vi "ComputeACPadPositions.vi"(0 "Theta Calibration":dbl format="%#_8g", 1 "X cp":dbl format="%#_8g", 2 "Y cp":dbl format="%#_8g", 3 "Stage Initial\nRotation":dbl, 4 "Sensor Path":path=path "R0Hamamatsu.txt ") -> ()   [LabVIEW 2018]
uses:
  <vilib>/Analysis/coordinate.llb/2D Cartesian Coordinate Rotation (Scalar).vi
  <vilib>/Utility/file.llb/Read Delimited Spreadsheet (DBL).vi
  <vilib>/Utility/file.llb/Write Delimited Spreadsheet (DBL).vi
  <vilib>/Analysis/NI_AALPro.lvlib
panel:
  out "error out":errorcluster
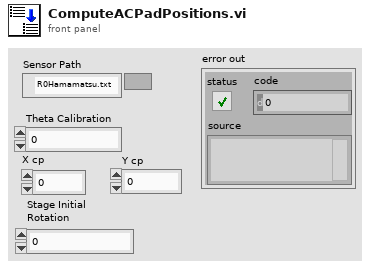
[diagram p1: front panel]
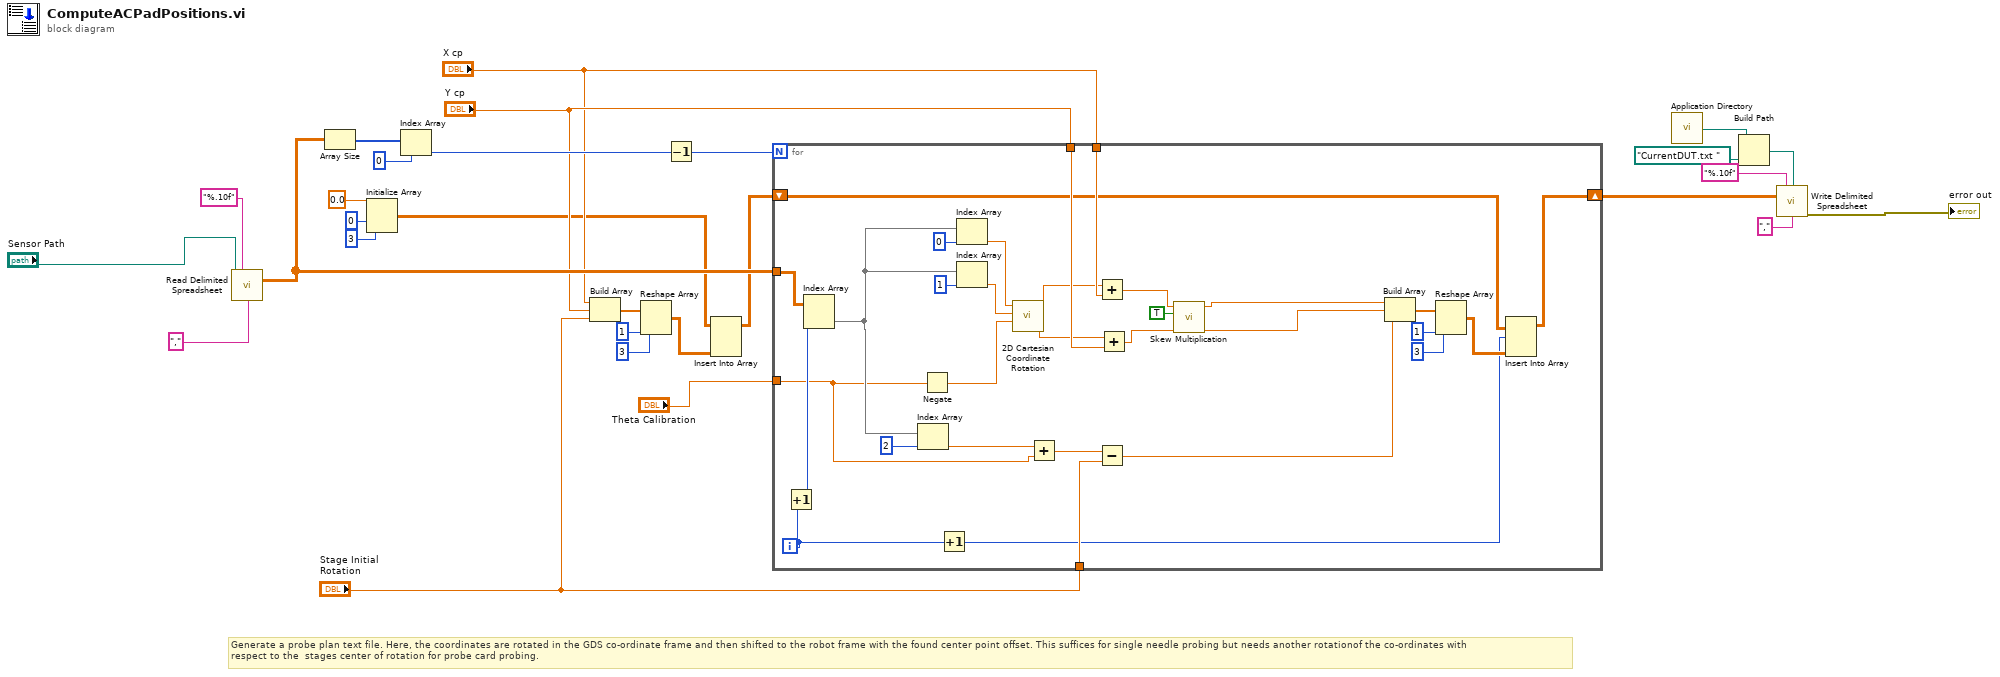
[diagram p0: block diagram]
diagram:
  # "Generate a probe plan text file. Here, the coordinates are rotated in the GDS co-ordinate frame and then shifted to the robot frame with the found center point offset. This suffices for single needle probing but needs another rotationof the co-ordinates with\nrespect to the  stages center of rotation for probe card probing."
  n1 = call-poly <vilib>:"Read Delimited Spreadsheet.vi"("file path (dialog if empty)"="Sensor Path", "format (%.3f)"="%.10f", "delimiter (\\t)"="," ("delimiter (\\t)")) -> ("all rows"=w25:dbl[][])  [unwired: 7 in, 5 out]
  n2 = Array Size(array=w25) -> (size(s)=w27:i32[])
  n3 = Initialize Array(0.0 ("element"), 0 ("dimension size"), 3 ("dimension size")) -> (w3:dbl[][])
  n4 = Index Array(array=w27, index=0) -> (element=w23:i32)
  n5 = Build Array("X cp", "Y cp", "Stage Initial\nRotation") -> (w10:dbl[])
  n6 = Reshape Array(w10, 1 ("dimension size"), 3 ("dimension size")) -> (w7:dbl[][])
  n7 = Decrement(x=w23) -> (x-1=w1:i32)
  n8 = Insert Into Array(array=w3, new element=w7) -> (w2:dbl[][])  [unwired: 2 in]
  n9 = for {
    N: w1 -> [_]
    tunnel: w25 -> [w59]
    tunnel: "Theta Calibration" -> [w31]
    tunnel: "X cp" -> [w54]
    tunnel: "Y cp" -> [w53]
    tunnel: "Stage Initial\nRotation" -> [w50]
    shift-right: [w44] -> w16
    shift-left: w2 -> [w45]
    i -> [w42]
    n10 = Increment(x=w42) -> (x+1=w32:i32)
    n11 = Index Array(array=w59, index (row)=w32) -> (element=w58:dbl[])  [unwired: 1 in]
    n12 = Index Array(array=w58, index=2) -> (element=w52:dbl)
    n13 = Negate(x=w31) -> (-x=w30:dbl)
    n14 = Increment(x=w42) -> (x+1=w29:i32)
    n15 = Index Array(array=w58, index=0) -> (element=w39:dbl)
    n16 = Index Array(array=w58, index=1) -> (element=w38:dbl)
    n17 = call-poly <vilib>:"2D Cartesian Coordinate Rotation.vi"("theta"=w30, "y"=w38, "x"=w39) -> ("y out"=w40:dbl, "x out"=w41:dbl)  [unwired: 6 in, 1 out]
    n18 = Add(x=w52, y=w31) -> (x+y=w51:dbl)
    n19 = Add(x=w41, y=w54) -> (x+y=w36:dbl)
    n20 = Subtract(x=w51, y=w50) -> (x-y=w46:dbl)
    n21 = Add(x=w40, y=w53) -> (x+y=w35:dbl)
    n22 = call "Skew Multiplication.vi"("Y"=w35, "Boolean"=TRUE, "X"=w36) -> ("Y'"=w33:dbl, "X'"=w34:dbl)  [unwired: 7 in]
    n23 = Build Array(w34, w33, w46) -> (w49:dbl[])
    n24 = Reshape Array(w49, 1 ("dimension size"), 3 ("dimension size")) -> (w43:dbl[][])
    n25 = Insert Into Array(array=w45, index (row)=w29, new element=w43) -> (w44:dbl[][])  [unwired: 1 in]
  }
  n26 = call <vilib>:"Application Directory.vi"() -> ("Application Directory"=w18:path)
  n27 = Build Path(base path=w18, name or relative path=path "CurrentDUT.txt " ("file path (dialog if empty)")) -> (appended path=w17:path)
  n28 = call-poly <vilib>:"Write Delimited Spreadsheet.vi"("file path (dialog if empty)"=w17, "format (%.3f)"="%.10f", "2D data"=w16, "delimiter (\\t)"="," ("delimiter (\\t)")) -> ("error out"=→"error out":errorcluster)  [unwired: 10 in, 1 out]
